vi "ex8-1.vi"   [LabVIEW 2009]
uses:
  <vilib>/NXT/Dual Mode Library/Sound/PlayD.vi
  <vilib>/NXT/Dual Mode Library/Sound/Tone.vi
types:
  T1 = typedef "LVHSConnector.ctl" = cluster{"error":errorcluster, "address":string, "NXT #":i32, "Show Error":bool, "Connection":u16}
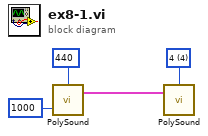
[diagram p0: block diagram]
diagram:
  w1 = u16 4 items=["3"=3, "4"=4, "5"=5, "6"=6, "7"=7] ("Octave")
  n1 = call-poly <vilib>:"PolySound.vi"("Duration (500 ms)"=u16 1000, "Tone (440 Hz)"=u16 440) -> ("NXT"=w4:T1)  [unwired: 2 in]
  n2 = call-poly <vilib>:"PolySound.vi"("NXT"=w4, "Octave"=w1) -> ()  [unwired: 2 in, 1 out]
